vi "Cache-BroadcastReg Search Result.vi"(8 "error in (no error)":errorcluster, 10 "JKISM Name":string, 11 "Broadcast state":string) -> (0 "error out":errorcluster, 3 "Array":T1(array[cluster]))   [LabVIEW 2014, in "JKI-State-Machine-Plus.lvlib"]
uses:
  JKI-State-Machine-Plus.lvlib
  JKISMQ/_JKISMQFGVOPER.ctl
  Oper-BroadcastRegistry.ctl
  global-BroadcastCacheChangeTStamp.vi
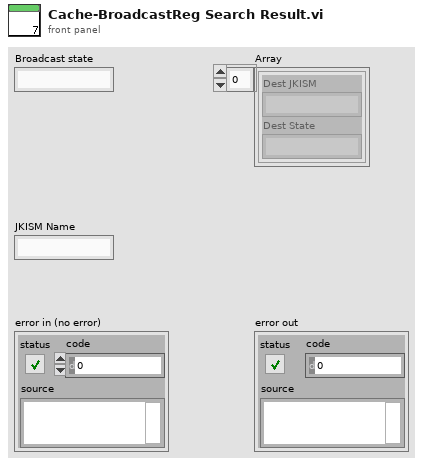
[diagram p1: front panel]
types:
  T1 = cluster{"Dest JKISM":string, "Dest State":string}[]
  T2 = cluster{"Dest JKISM":string, "Dest State":string}
  T3 = typedef "JKI-State-Machine-Plus.lvlib/_JKISMQFGVOPER.ctl" = enum16{"Get By Name", "List", "Check If Name Exists", "Release"}
  T4 = typedef "JKI-State-Machine-Plus.lvlib/Oper-BroadcastRegistry.ctl" = enum16{"Delete Source Module", "Delete Dest Module", "Remove Module", "Register", "Unregister", "Check"}
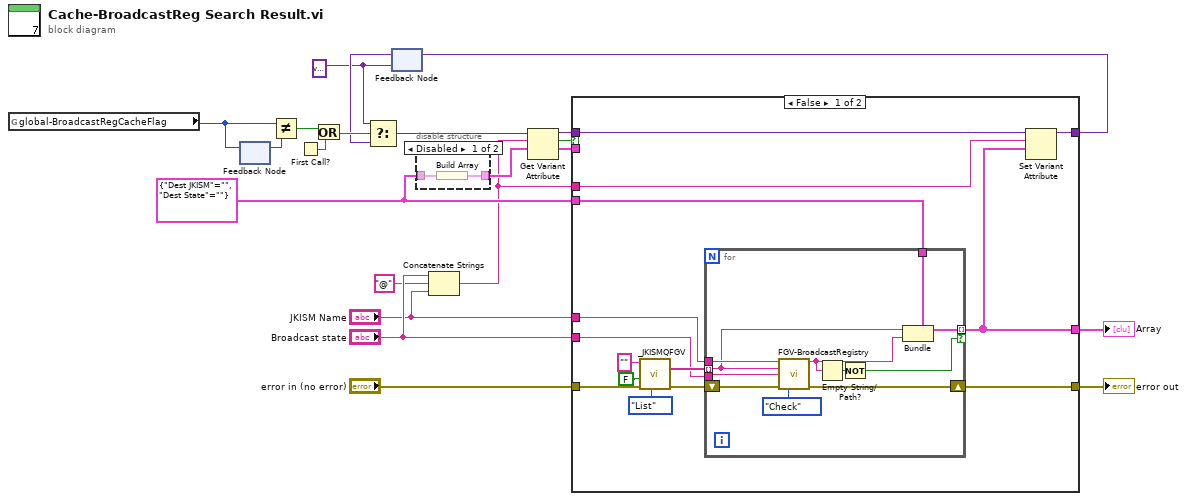
[diagram p0: block diagram]
diagram:
  w9 = T2 {"Dest JKISM"="", "Dest State"=""} ("cluster")
  w14 = variant
  n1 = global read "global-BroadcastCacheChangeTStamp.vi" "global-BroadcastRegCacheFlag"() -> (w2:u32)
  n2 = feedback-in #1(w2) -> ()
  n3 = feedback #1() -> (w1:u32)  [unwired: 1 in]
  n4 = Not Equal?(x=w2, y=w1) -> (x != y?=w18:bool)
  n5 = First Call?() -> (First Call?: T/F=w17:bool)
  n6 = Or(x=w18, y=w17) -> (x .or. y?=w16:bool)
  n7 = feedback #2(w14) -> (w15:variant)
  n8 = Select(t=w14, s=w16, f=w15) -> (s? t:f=w10:variant)
  n9 = disable-structure shown="Disabled" {
    disable-tunnel: w9 -> [w23 _]
    disable-tunnel: [w22 _] -> w8
    frame Disabled {
      n10 = Build Array(w23) -> (w22:T1)
    }
    frame Enabled {
    }
  }
  n11 = Concatenate Strings("Broadcast state", "@" ("string"), "JKISM Name") -> (w4:string)
  n12 = Get Variant Attribute(Variant=w10, name=w4, default value (empty Variant)=w8) -> (duplicate Variant=w6:variant, found=w7:bool, value=w5:T1)  [unwired: 1 in, 1 out]
  n13 = case shown="False" w7 {
    tunnel: [w37 w50] -> w21
    tunnel: "error in (no error)" -> [w34 w50]
    tunnel: [w25 w51] -> w19
    tunnel: "Broadcast state" -> [w30 _]
    tunnel: "JKISM Name" -> [w29 _]
    tunnel: w9 -> [w28 _]
    tunnel: w6 -> [w27 w49]
    tunnel: w5 -> [_ w51]
    tunnel: w4 -> [w26 _]
    tunnel: [w24 w49] -> w3
    frame False {
      n14 = call "_JKISMQFGV.vi"(6:_JKISMQFGVOPER."List", "Error in"=w34, "create if not found? (T)"=FALSE, "Name(\"\" to use uuid) in"="" ("Name(\"\" to use uuid) in")) -> ("Error out"=w36:errorcluster, "Name"=w35:string[])  [unwired: 4 in, 2 out]
      n15 = for {
        tunnel: w35 -> [w43] mode=indexing
        tunnel: w29 -> [w46]
        tunnel: w30 -> [w41]
        shift-right: [w44] -> w37
        shift-left: w36 -> [w47]
        tunnel: [w40] -> w25 mode=indexing if=w42
        tunnel: w28 -> [w38]
        n16 = call "FGV-BroadcastRegistry.vi"("Source"=w46, "Dest"=w43, "Message"=w41, "Error in"=w47, "Operation"=Oper-BroadcastRegistry."Check") -> ("ActingMsg out"=w39:string, "Error out"=w44:errorcluster)  [unwired: 8 in, 1 out]
        n17 = Empty String/Path?(string/path=w39) -> (empty?=w45:bool)
        n18 = Not(x=w45) -> (.not. x?=w42:bool)
        n19 = Bundle(cluster=w38, "Dest JKISM"=w43, "Dest State"=w39) -> (w40:T2)
      }
      n20 = Set Variant Attribute(Variant=w27, name=w26, value=w25) -> (Variant out=w24:variant)  [unwired: 1 in, 2 out]
    }
    frame True {
    }
  }
  "error out" <- w21
  "Array" <- w19
  n21 = feedback-in #2(w3) -> ()
